vi "BKP_PowerSupplies1697B.vi"(4 "Error In":errorcluster, 7 "Command":T13) -> (0 "Error Out":errorcluster, 3 "Response":T11)   [LabVIEW 2018]
uses:
  MOKO_LabViewLibrary/MokoLowLevel/MokoLowLovelControl/MLLC_Command.ctl
  MOKO_LabViewLibrary/MokoLowLevel/MokoLowLovelControl/MLLC_Mode.ctl
  MOKO_LabViewLibrary/MokoLowLevel/MokoLowLovelControl/MLLC_Response.ctl
  MOKO_LabViewLibrary/MokoLowLevel/MokoLowLovelControl/MLLC_ConnectCluster.ctl
  MOKO_LabViewLibrary/MokoLowLevel/MokoLowLovelControl/MLLC_InterfaceType.ctl
  MOKO_LabViewLibrary/MokoLowLevel/MokoLowLovelControl/MLLC_OpenedSession.ctl
  MOKO_LabViewLibrary/MokoLowLevel/MokoLowLovelControl/MLLC_InterfaceSettings.ctl
  MOKO_LabViewLibrary/MokoLowLevel/MokoLowLovelControl/MLLC_InterfaceKind.ctl
  MOKO_LabViewLibrary/MokoLowLevel/MokoLowLovelControl/MLLC_DriverName.ctl
  MOKO_LabViewLibrary/MokoLowLevel/MokoLowLovelControl/MLLC_ResponseInit.ctl
  MOKO_LabViewLibrary/MokoLowLevel/MokoLowLovelControl/MLLC_Request.ctl
  MOKO_LabViewLibrary/MokoLowLevel/MokoLowLovelControl/MLLC_ErrorCode.ctl
  MOKO_LabViewLibrary/MokoLowLevel/MokoLowLovelControl/MLLC_Rs232Settings.ctl
panel:
  in  "Error Code":T1=5420
  in  "Request":T2="GETS"
  in  "ResponseInit":T3="OK"
  in  "Driver Name":T4="BK1697B"
  in  "Settings":T10={"Permanent data"={"Connect"={"InterfaceType"=enum."VISA", "OpenedSession"="", "InterfaceSettings"={"Interface"=enum."RS232", "EOS 4 read"=enum."CR (\\r)", "EOS 4 write"=enum."CR (\\r)", "TMO, ms"=2000, "Sett"=variant(cluster{"Baud Rate":u32, "Data Bits":u16, "Parity":u16, "Stop Bits":u16, "Flow Control":u16, "Eho":bool} {"Baud Rate"=75, "Data Bits"=0, "Parity"=0, "Stop Bits"=0, "Flow Control"=0, "Eho"=FALSE})}}}, "Saved Data"=variant}
  in  "Mode":T12=enum."Check"
  # "BK1697B"
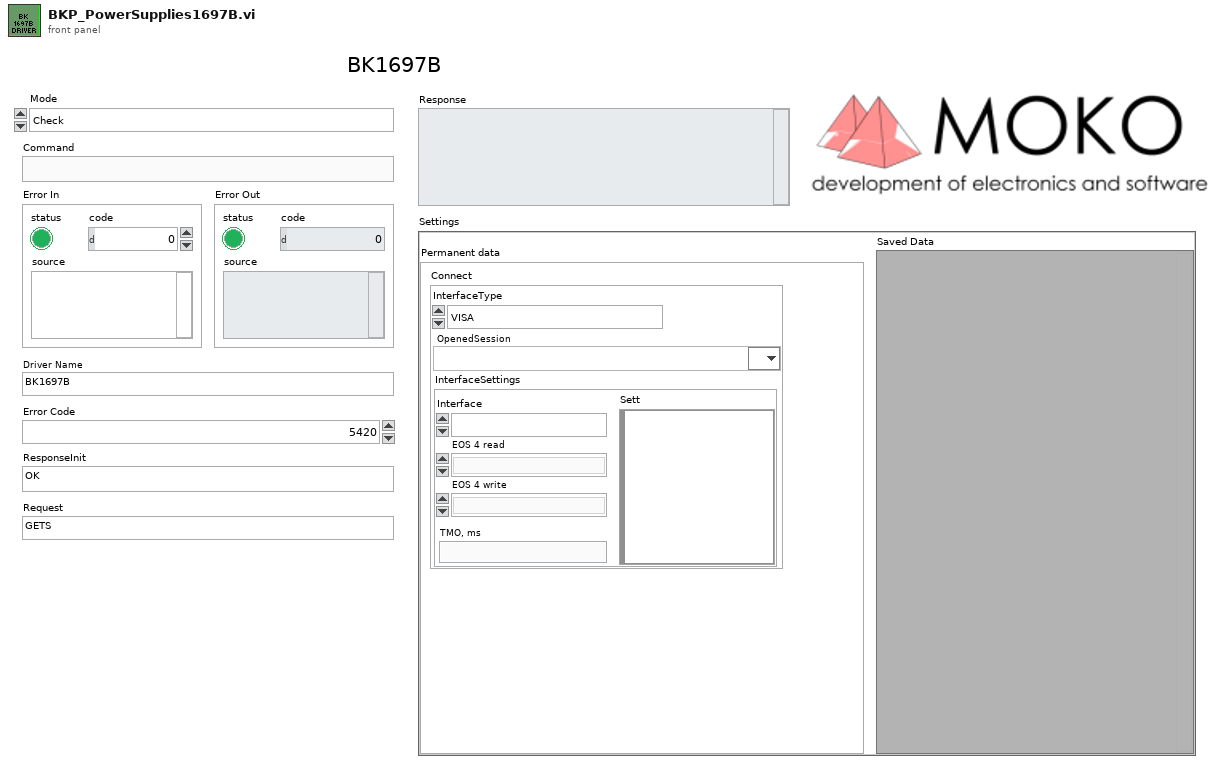
[diagram p1: front panel]
types:
  T1 = typedef "MLLC_ErrorCode.ctl" = u32
  T2 = typedef "MLLC_Request.ctl" = string
  T3 = typedef "MLLC_ResponseInit.ctl" = string
  T4 = typedef "MLLC_DriverName.ctl" = string
  T5 = typedef "MLLC_ConnectCluster.ctl" = cluster{"InterfaceType":T6, "OpenedSession":T7, "InterfaceSettings":T8}
  T6 = typedef "MLLC_InterfaceType.ctl" = enum16{"VISA", "Prologix USB-GPIB"}
  T7 = typedef "MLLC_OpenedSession.ctl" = refnum<visa-resource-name>
  T8 = typedef "MLLC_InterfaceSettings.ctl" = cluster{"Interface":T9, "EOS 4 read":enum16{"Default (=EOS 4 write)", "CR (\\r)", "LF (\\n)", "None"}, "EOS 4 write":enum16{"CR+LF (\\r\\n)", "CR (\\r)", "LF (\\n)", "None"}, "TMO, ms":i32, "Sett":variant}
  T9 = typedef "MLLC_InterfaceKind.ctl" = enum16{"RS232", "GPIB", "USB", "Ethernet", "another"}
  T10 = cluster{"Permanent data":cluster{"Connect":T5}, "Saved Data":variant}
  T11 = typedef "MLLC_Response.ctl" = string
  T12 = typedef "MLLC_Mode.ctl" = enum16{"get", "set", "close", "Init", "Check"}
  T13 = typedef "MLLC_Command.ctl" = string
  T14 = typedef "MLLC_Error.ctl" = errorcluster
  T15 = typedef "MLLC_Rs232Settings.ctl" = cluster{"Baud Rate":u32, "Data Bits":u16, "Parity":u16, "Stop Bits":u16, "Flow Control":u16, "Eho":bool, "Address":dbl}
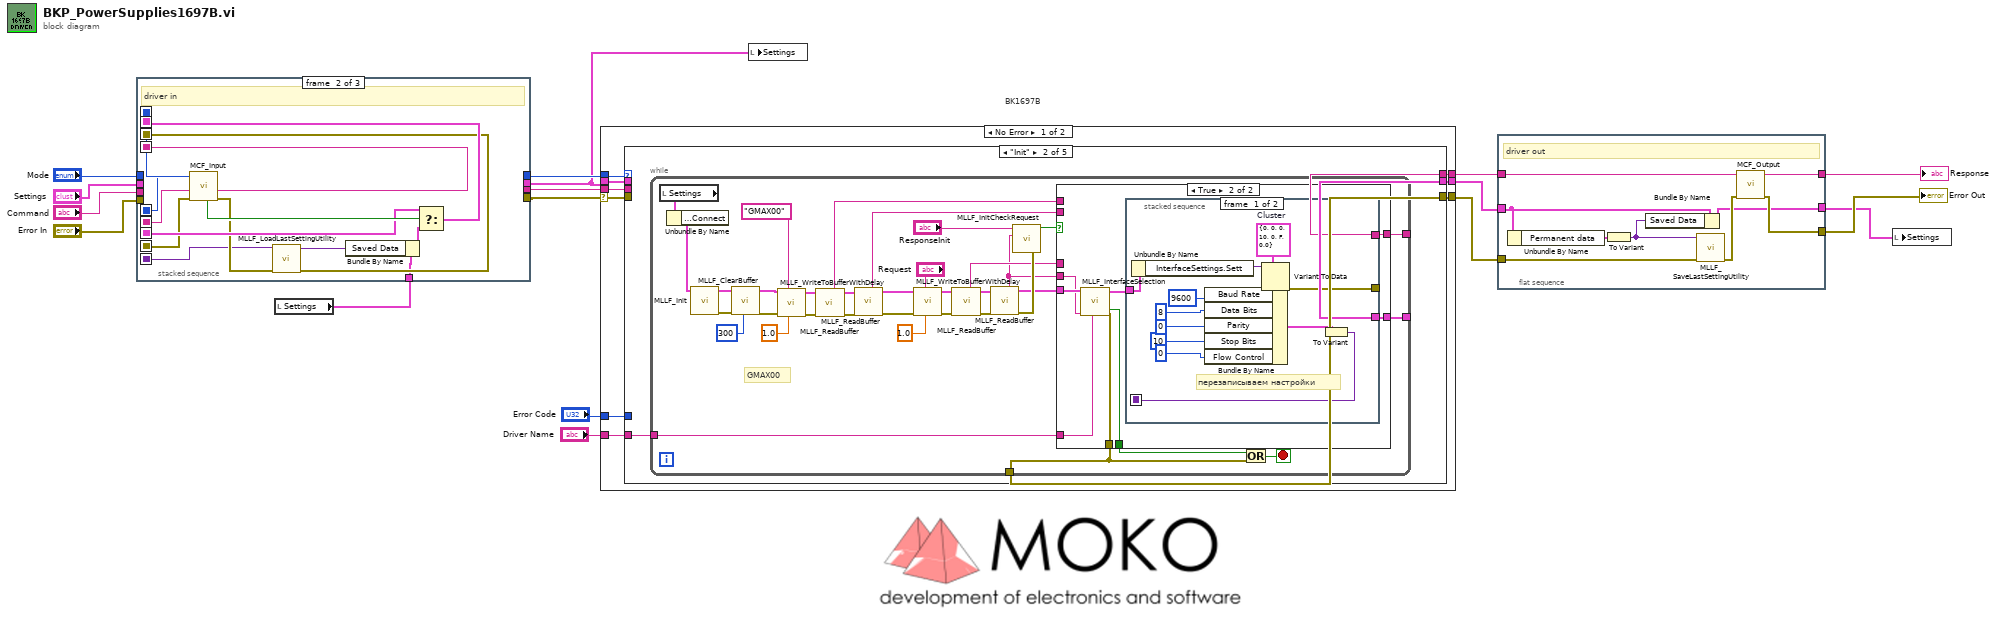
[diagram p0: block diagram]
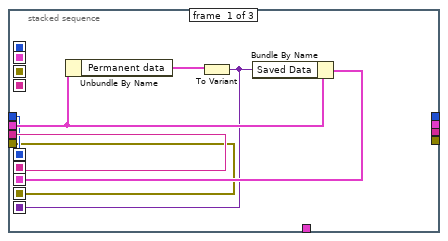
[diagram p2: hidden frame]
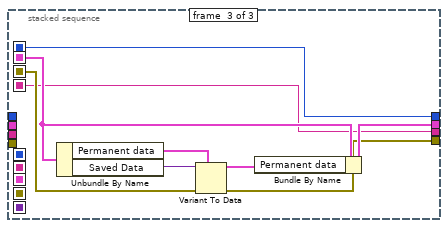
[diagram p3: hidden frame]
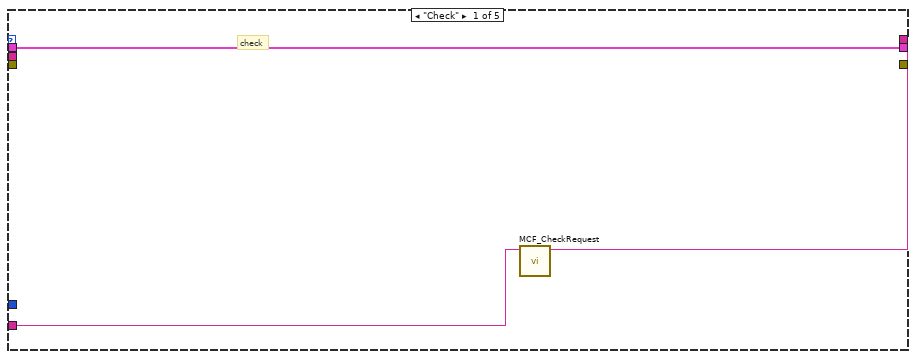
[diagram p4: hidden frame]
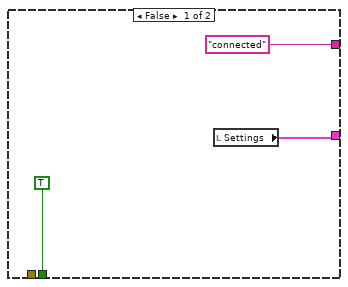
[diagram p5: hidden frame]
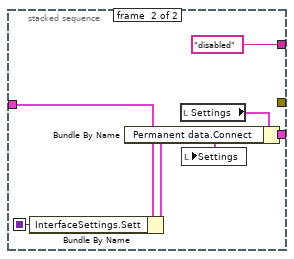
[diagram p6: hidden frame]
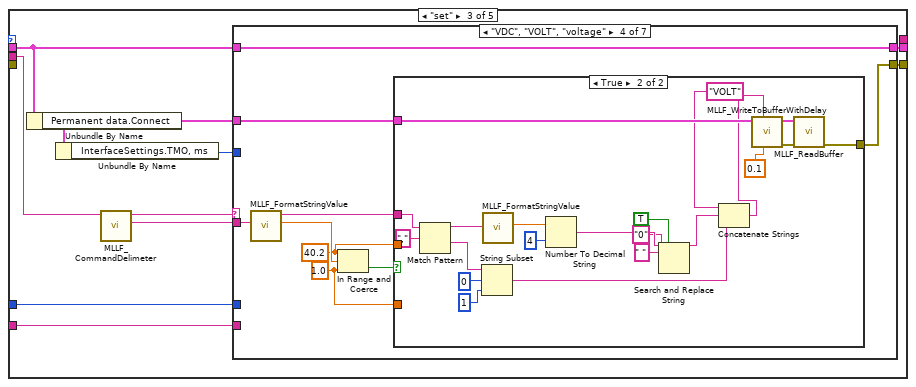
[diagram p7: hidden frame]
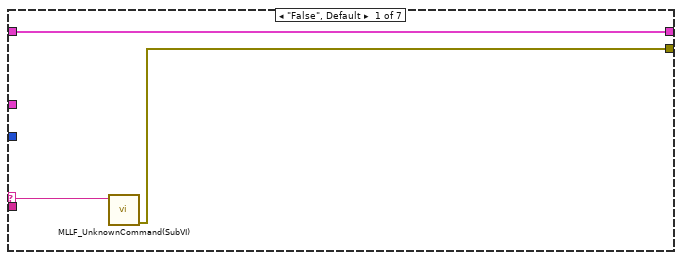
[diagram p8: hidden frame]
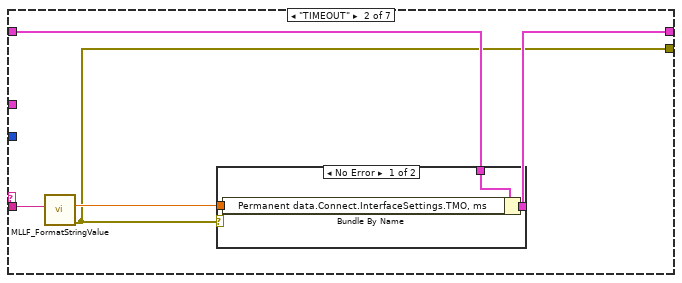
[diagram p9: hidden frame]
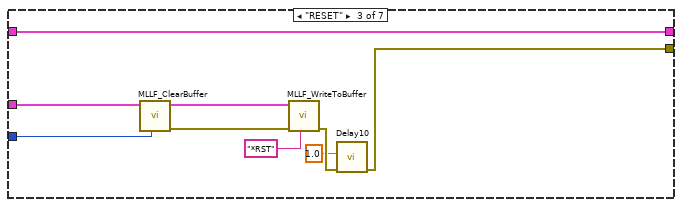
[diagram p11: hidden frame]
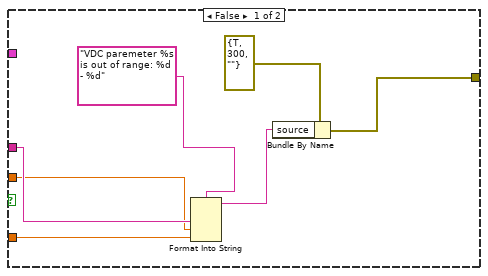
[diagram p12: hidden frame]
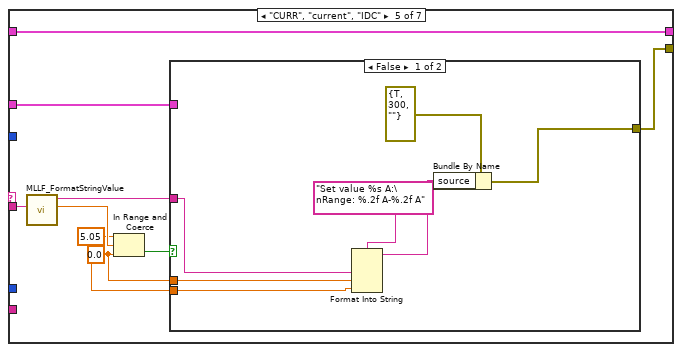
[diagram p13: hidden frame]
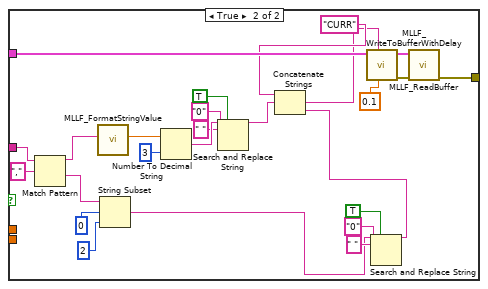
[diagram p14: hidden frame]
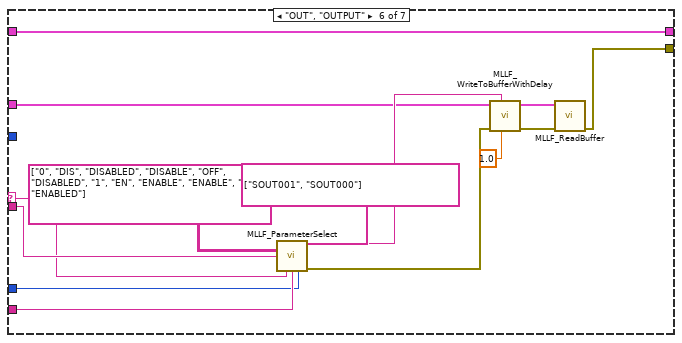
[diagram p15: hidden frame]
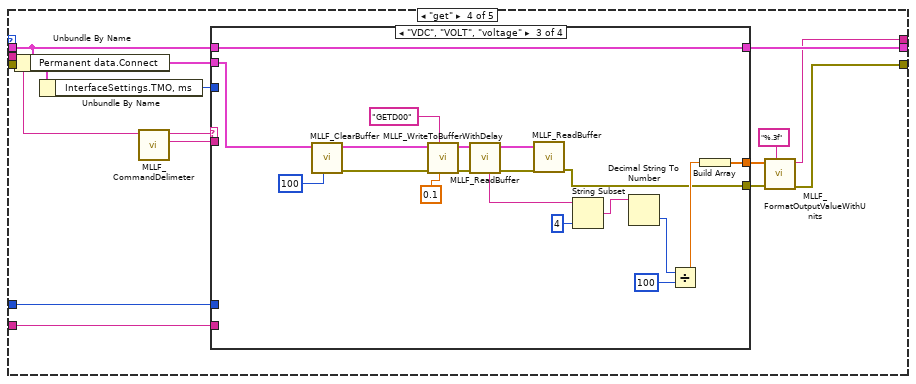
[diagram p17: hidden frame]
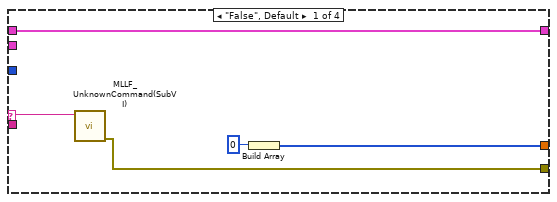
[diagram p18: hidden frame]
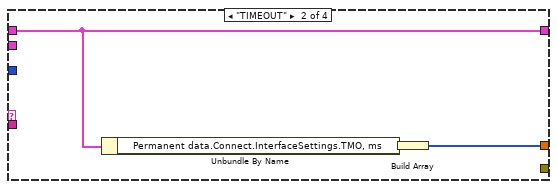
[diagram p19: hidden frame]
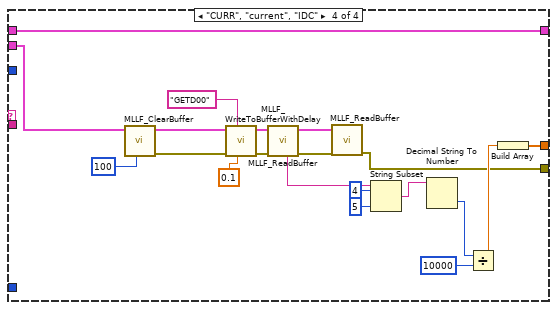
[diagram p20: hidden frame]
diagram:
  # "BK1697B"
  n1 = local read "Settings"() -> (w8:T10)
  n2 = stacked-sequence {
    seq-local: [w20 _ _] -> [_ w36 _]
    seq-local: [w19 _ _] -> [_ w37 _]
    seq-local: [w22 _ _] -> [_ w32 _]
    seq-local: [w18 _ _] -> [_ w31 _]
    seq-local: [w21 _ _] -> [_ w27 _]
    seq-local: [_ w28 _] -> [_ _ w44]
    seq-local: [_ w38 _] -> [_ _ w41]
    seq-local: [_ w35 _] -> [_ _ w40]
    seq-local: [_ w34 _] -> [_ _ w45]
    tunnel: "Command" -> [w20 _ _]
    tunnel: "Mode" -> [w19 _ _]
    tunnel: "Error In" -> [w18 _ _]
    tunnel: "Settings" -> [w23 _ _]
    tunnel: w8 -> [_ w26 _]
    tunnel: [_ _ w40] -> w10
    tunnel: [_ _ w43] -> w1
    tunnel: [_ _ w42] -> w9
    tunnel: [_ _ w41] -> w11
    frame #0 {
      n3 = Unbundle By Name(w23) -> ("Permanent data"=w24:cluster{"Connect":T5})
      n4 = To Variant(anything=w24) -> (Variant=w21:variant)
      n5 = Bundle By Name(cluster=w23, "Saved Data"=w21) -> (w22:T10)
    }
    frame #1 {
      # "driver in"
      n6 = call "MCF_Input.vi"("Error In"=w31, "Command in"=w36, "Mode in"=w37) -> ("Error Out"=w30:errorcluster, "Command out"=w35:string, "Mode out"=w38:T12, "Boolean"=w33:bool)  [unwired: 5 in]
      n7 = call "MLLF_LoadLastSettingUtility.vi"("Error In"=w30, "Save data in"=w27) -> ("Error Out"=w28:errorcluster, "Save data out"=w25:variant)  [unwired: 8 in]
      n8 = Bundle By Name(cluster=w26, "Saved Data"=w25) -> (w29:T10)
      n9 = Select(t=w32, s=w33, f=w29) -> (s? t:f=w34:T10)
    }
    frame #2 {
      n10 = Unbundle By Name(w45) -> ("Permanent data"=w46:cluster{"Connect":T5}, "Saved Data"=w39:variant)
      n11 = Variant To Data(error in=w44, type=w46, Variant=w39) -> (data=w47:cluster{"Connect":T5}, error out=w42:errorcluster)
      n12 = Bundle By Name(cluster=w45, "Permanent data"=w47) -> (w43:T10)
    }
  }
  n13 = case shown="No Error" w9 {
    selector: w9 -> [w52 w318]
    tunnel: [w54 w318] -> w5
    tunnel: w11 -> [w56 _]
    tunnel: [w55 _] -> w7
    tunnel: w10 -> [w53 _]
    tunnel: w1 -> [w49 w317]
    tunnel: "Error Code" -> [w51 _]
    tunnel: "Driver Name" -> [w50 _]
    tunnel: [w48 w317] -> w6
    frame No Error {
      n14 = case shown="\"Init\"" w56 {
        tunnel: [w57 w61 _ w253 "" ("Output String")] -> w55
        tunnel: [_ w63 w131 w254 w315] -> w54
        tunnel: w53 -> [_ _ w130 w259 _]
        tunnel: w52 -> [_ _ _ _ _]
        tunnel: w51 -> [_ _ w137 w263 _]
        tunnel: w50 -> [w58 w60 w134 w262 _]
        tunnel: w49 -> [w59 _ w136 w265 w314]
        tunnel: [w59 w62 w135 w264 w314] -> w48
        frame "Check" {
          # "check"
          n15 = call "MCF_CheckRequest.vi"("Driver Name"=w58) -> ("Output String"=w57:string)  [unwired: 9 in, 1 out]
        }
        frame "Init" {
          n16 = while {
            tunnel: [w92] -> w63
            tunnel: [w89] -> w62
            tunnel: [w88] -> w61
            tunnel: w60 -> [w77]
            stop <- w94 stop-if-true
            # "GMAX00"
            n17 = local read "Settings"() -> (w98:T10)
            n18 = Unbundle By Name(w98) -> ("Permanent data.Connect"=w95:T5)
            n19 = call "MLLF_Init.vi"("DriverConnect in"=w95) -> ("Error Out"=w80:errorcluster, "DriverConnect out"=w81:T5)  [unwired: 7 in]
            n20 = call "MLLF_ClearBuffer.vi"("Timeout(default = 300 ms)"=u32 300 ("Timeout"), "Error In"=w80, "DriverConnect in"=w81) -> ("Error Out"=w69:errorcluster, "DriverConnect out"=w70:T5)  [unwired: 5 in, 1 out]
            n21 = call "MLLF_WriteToBufferWithDelay.vi"("Delay Time ( 0,05 s)"=1.0 ("Delay Time (s)"), "Command"=T2 "GMAX00" ("Request 2"), "Error In"=w69, "DriverConnect in"=w70) -> ("Error Out"=w74:errorcluster, "DriverConnect out"=w72:T5)  [unwired: 6 in]
            n22 = call "MLLF_ReadBuffer.vi"("Error In"=w74, "DriverConnect in"=w72) -> ("Error Out"=w76:errorcluster, "DriverConnect out"=w75:T5, "String"=w66:string)  [unwired: 6 in]
            n23 = call "MLLF_ReadBuffer.vi"("Error In"=w76, "DriverConnect in"=w75) -> ("Error Out"=w67:errorcluster, "DriverConnect out"=w68:T5, "String"=w65:string)  [unwired: 6 in]
            n24 = call "MLLF_WriteToBufferWithDelay.vi"("Delay Time ( 0,05 s)"=1.0 ("Delay Time (s)"), "Command"="Request", "Error In"=w67, "DriverConnect in"=w68) -> ("Error Out"=w91:errorcluster, "DriverConnect out"=w97:T5)  [unwired: 6 in]
            n25 = call "MLLF_ReadBuffer.vi"("Error In"=w91, "DriverConnect in"=w97) -> ("Error Out"=w84:errorcluster, "DriverConnect out"=w85:T5, "String"=w78:string)  [unwired: 6 in]
            n26 = call "MLLF_ReadBuffer.vi"("Error In"=w84, "DriverConnect in"=w85) -> ("Error Out"=w83:errorcluster, "DriverConnect out"=w82:T5, "String"=w64:string)  [unwired: 6 in]
            n27 = call "MLLF_InitCheckRequest.vi"("error in (no error)"=w83, "Answer"=w64, "Response Init"="ResponseInit") -> ("Design"=w86:bool)  [unwired: 5 in, 3 out]
            n28 = case shown="True" w86 {
              tunnel: w82 -> [_ w108]
              tunnel: [TRUE w104] -> w93
              tunnel: [_ w109] -> w92
              tunnel: [w99 w106] -> w89
              tunnel: ["connected" w105] -> w88
              tunnel: w78 -> [_ _]
              tunnel: w77 -> [_ w103]
              tunnel: w66 -> [_ _]
              tunnel: w65 -> [_ _]
              tunnel: w64 -> [_ w102]
              frame False {
                n29 = local read "Settings"() -> (w99:T10)
              }
              frame True {
                n30 = call "MLLF_InterfaceSelection.vi"("Driver Name"=w103, "Answer:"=w102, "DriverConnect in"=w108) -> ("error out"=w109:T14, "DriverConnect out"=w107:T5, "stop init?"=w104:bool)  [unwired: 4 in, 2 out]
                n31 = stacked-sequence {
                  seq-local: [w112 _] -> [_ w126]
                  tunnel: w107 -> [w111 w123]
                  tunnel: [w113 _] -> _
                  tunnel: [_ w125] -> w106
                  tunnel: [_ "disabled"] -> w105
                  frame #0 {
                    w115 = T15 {"Baud Rate"=0, "Data Bits"=0, "Parity"=0, "Stop Bits"=10, "Flow Control"=0, "Eho"=FALSE, "Address"=0.0}  # Cluster
                    # "перезаписываем настройки"
                    n32 = Unbundle By Name(w111) -> ("InterfaceSettings.Sett"=w114:variant)
                    n33 = Variant To Data(type=w115, Variant=w114) -> (data=w116:T15, error out=w113:errorcluster)  [unwired: 1 in]
                    n34 = Bundle By Name(cluster=w116, "Baud Rate"=u32 9600, "Data Bits"=u16 8 ("Serial Settings:Data Bits"), "Parity"=u16 0 ("Serial Settings:Parity"), "Stop Bits"=u16 10 ("Serial Settings:Stop Bits"), "Flow Control"=u16 0 ("Serial Settings:Flow Control")) -> (w121:T15)
                    n35 = To Variant(anything=w121) -> (Variant=w112:variant)
                  }
                  frame #1 {
                    n36 = Bundle By Name(cluster=w123, "InterfaceSettings.Sett"=w126) -> (w122:T5)
                    n37 = local read "Settings"() -> (w127:T10)
                    n38 = Bundle By Name(cluster=w127, "Permanent data.Connect"=w122) -> (w125:T10)
                    n39 = local write "Settings"(w125) -> ()
                  }
                }
              }
            }
            n40 = Or(x=w93, y=w92) -> (x .or. y?=w94:bool)
          }
        }
        frame "set" {
          n41 = Unbundle By Name(w136) -> ("Permanent data.Connect"=w133:T5)
          n42 = Unbundle By Name(w133) -> ("InterfaceSettings.TMO, ms"=w132:i32)
          n43 = call "MLLF_CommandDelimeter.vi"("command with param"=w130) -> ("param 1"=w128:string, "command"=w129:string)  [unwired: 6 in, 3 out]
          n44 = case shown="\"VDC\", \"VOLT\", \"voltage\"" w129 {
            selector: w129 -> [w139 _ _ _ _ w240 _]
            tunnel: w128 -> [_ w143 _ w166 w203 w249 _]
            tunnel: w137 -> [_ _ _ _ _ w245 _]
            tunnel: w136 -> [w140 w144 w158 w167 w204 w250 w251]
            tunnel: [w140 w145 w158 w167 w204 w250 w251] -> w135
            tunnel: w133 -> [_ _ w156 w165 w202 w241 _]
            tunnel: w134 -> [_ _ _ _ _ w246 _]
            tunnel: w132 -> [_ _ w153 _ _ _ _]
            tunnel: [w138 w141 w150 w164 w201 w237 _] -> w131
            frame "False", Default {
              n45 = call "MLLF_UnknownCommand(SubVI).vi"("Unknown command"=w139) -> ("error out"=w138:errorcluster)  [unwired: 10 in]
            }
            frame "TIMEOUT" {
              n46 = call "MLLF_FormatStringValue.vi"("String Value"=w143) -> ("error out"=w141:T14, "number"=w142:dbl)  [unwired: 8 in, 1 out]
              n47 = case shown="No Error" w141 {
                tunnel: [w148 w149] -> w145
                tunnel: w144 -> [w147 w149]
                tunnel: w142 -> [w146 _]
                frame No Error {
                  n48 = Bundle By Name(cluster=w147, "Permanent data.Connect.InterfaceSettings.TMO, ms"=w146) -> (w148:T10)
                }
                frame Error {
                }
              }
            }
            frame "RESET" {
              n49 = call "MLLF_ClearBuffer.vi"("Timeout(default = 300 ms)"=w153, "DriverConnect in"=w156) -> ("Error Out"=w155:errorcluster, "DriverConnect out"=w154:T5)  [unwired: 6 in, 1 out]
              n50 = call "MLLF_WriteToBuffer.vi"("String"="*RST", "error in"=w155, "DriverConnect in"=w154) -> ("error out"=w152:T14)  [unwired: 5 in, 1 out]
              n51 = call "Delay10"("error in (no error)"=w152, "Delay Time (s)"=1.0) -> ("error out"=w150:errorcluster)  [unwired: 9 in]
            }
            frame "VDC", "VOLT", "voltage" {
              w160 = 1.0 ("lower limit")
              w159 = 40.2 ("upper limit")
              n52 = call "MLLF_FormatStringValue.vi"("String Value"=w166) -> ("number"=w162:dbl, "String Value Formated"=w163:T13)  [unwired: 8 in, 1 out]
              n53 = In Range and Coerce(upper limit=w159, x=w162, lower limit=w160) -> (In Range?=w161:bool)  [unwired: 1 out]
              n54 = case shown="True" w161 {
                tunnel: w165 -> [_ w192]
                tunnel: [w173 w191] -> w164
                tunnel: w163 -> [w172 w188]
                tunnel: w160 -> [w169 _]
                tunnel: w159 -> [w168 _]
                frame False {
                  n55 = Format Into String(format string="VDC paremeter %s is out of range: %d - %d", w172, w168, w169) -> (resulting string=w171:string)  [unwired: 2 in, 1 out]
                  n56 = Bundle By Name(cluster=errorcluster {"status"=TRUE, "code"=300, "source"=""} ("Error Out"), "source"=w171) -> (w173:errorcluster)
                }
                frame True {
                  n57 = Match Pattern(string=w188, regular expression=",") -> (before substring=w180:T13, after substring=w186:T13)  [unwired: 1 in, 2 out]
                  n58 = String Subset(string=w186, offset (0)=0, length (rest)=1 ("length (rest)")) -> (substring=w183:T13)
                  n59 = call "MLLF_FormatStringValue.vi"("String Value"=w180) -> ("number"=w182:dbl)  [unwired: 8 in, 2 out]
                  n60 = Number To Decimal String(number=w182, width (-)=i16 4) -> (decimal integer string=w179:string)
                  n61 = Search and Replace String(replace all?=TRUE ("replace all? (F)"), input string=w179, search string=" ", replace string="0" ("replace string (\"\")")) -> (result string=w176:string)  [unwired: 4 in, 3 out]
                  n62 = Concatenate Strings(T13 "VOLT" ("Command"), w176, w183) -> (w189:string)
                  n63 = call "MLLF_WriteToBufferWithDelay.vi"("Delay Time ( 0,05 s)"=0.1 ("Delay Time (s)"), "Command"=w189, "DriverConnect in"=w192) -> ("Error Out"=w194:errorcluster, "DriverConnect out"=w195:T5)  [unwired: 7 in]
                  n64 = call "MLLF_ReadBuffer.vi"("Error In"=w194, "DriverConnect in"=w195) -> ("Error Out"=w191:errorcluster)  [unwired: 6 in, 2 out]
                }
              }
            }
            frame "CURR", "current", "IDC" {
              w197 = 0.0 ("lower limit")
              w196 = 5.05 ("upper limit")
              n65 = call "MLLF_FormatStringValue.vi"("String Value"=w203) -> ("number"=w199:dbl, "String Value Formated"=w200:T13)  [unwired: 8 in, 1 out]
              n66 = In Range and Coerce(upper limit=w196, x=w199, lower limit=w197) -> (In Range?=w198:bool)  [unwired: 1 out]
              n67 = case shown="False" w198 {
                tunnel: w202 -> [_ w233]
                tunnel: [w210 w232] -> w201
                tunnel: w200 -> [w208 w229]
                tunnel: w197 -> [w206 _]
                tunnel: w196 -> [w205 _]
                frame False {
                  n68 = Format Into String(format string="Set value %s A:\nRange: %.2f A-%.2f A", w208, w206, w205) -> (resulting string=w207:string)  [unwired: 2 in, 1 out]
                  n69 = Bundle By Name(cluster=errorcluster {"status"=TRUE, "code"=300, "source"=""} ("Error Out"), "source"=w207) -> (w210:errorcluster)
                }
                frame True {
                  n70 = Match Pattern(string=w229, regular expression=",") -> (before substring=w222:T13, after substring=w227:T13)  [unwired: 1 in, 2 out]
                  n71 = call "MLLF_FormatStringValue.vi"("String Value"=w222) -> ("number"=w224:dbl)  [unwired: 8 in, 2 out]
                  n72 = String Subset(string=w227, offset (0)=0, length (rest)=2 ("length (rest)")) -> (substring=w213:T13)
                  n73 = Number To Decimal String(number=w224, width (-)=i16 3) -> (decimal integer string=w221:string)
                  n74 = Search and Replace String(replace all?=TRUE ("replace all? (F)"), input string=w221, search string=" ", replace string="0" ("replace string (\"\")")) -> (result string=w218:string)  [unwired: 4 in, 3 out]
                  n75 = Search and Replace String(replace all?=TRUE ("replace all? (F)"), input string=w213, search string=" ", replace string="0" ("replace string (\"\")")) -> (result string=w212:string)  [unwired: 4 in, 3 out]
                  n76 = Concatenate Strings(T13 "CURR" ("Command"), w218, w212) -> (w230:string)
                  n77 = call "MLLF_WriteToBufferWithDelay.vi"("Delay Time ( 0,05 s)"=0.1 ("Delay Time (s)"), "Command"=w230, "DriverConnect in"=w233) -> ("Error Out"=w235:errorcluster, "DriverConnect out"=w236:T5)  [unwired: 7 in]
                  n78 = call "MLLF_ReadBuffer.vi"("Error In"=w235, "DriverConnect in"=w236) -> ("Error Out"=w232:errorcluster)  [unwired: 6 in, 2 out]
                }
              }
            }
            frame "OUT", "OUTPUT" {
              n79 = call "MLLF_ParameterSelect.vi"("Command to equipment"=string[] ["SOUT001", "SOUT000"] ("Names"), "Names"=string[][] [["0", "DIS", "DISABLED", "DISABLE", "OFF", "DISABLED"], ["1", "EN", "ENABLE", "ENABLE", "ON", "ENABLED"]], "Input"=w249, "Command"=w240, "Driver Name"=w246, "Error Code"=w245) -> ("Choice"=w242:string, "Error Out"=w243:errorcluster)  [unwired: 8 in]
              n80 = call "MLLF_WriteToBufferWithDelay.vi"("Delay Time ( 0,05 s)"=1.0 ("Delay Time (s)"), "Command"=w242, "Error In"=w243, "DriverConnect in"=w241) -> ("Error Out"=w239:errorcluster, "DriverConnect out"=w238:T5)  [unwired: 6 in]
              n81 = call "MLLF_ReadBuffer.vi"("Error In"=w239, "DriverConnect in"=w238) -> ("Error Out"=w237:errorcluster)  [unwired: 6 in, 2 out]
            }
            frame "****************************************************" {
            }
          }
        }
        frame "get" {
          n82 = Unbundle By Name(w265) -> ("Permanent data.Connect"=w256:T5)
          n83 = Unbundle By Name(w256) -> ("InterfaceSettings.TMO, ms"=w255:i32)
          n84 = call "MLLF_CommandDelimeter.vi"("command with param"=w259) -> ("param 1"=w257:string, "command"=w258:string)  [unwired: 6 in, 3 out]
          n85 = case shown="\"VDC\", \"VOLT\", \"voltage\"" w258 {
            selector: w258 -> [w267 _ _ _]
            tunnel: w257 -> [_ _ _ _]
            tunnel: [w266 _ w278 w298] -> w261
            tunnel: w263 -> [_ _ _ _]
            tunnel: [w270 w273 w292 w312] -> w264
            tunnel: w265 -> [w270 w273 w292 w312]
            tunnel: [w268 w271 w281 w301] -> w260
            tunnel: w256 -> [_ _ w276 w296]
            tunnel: w262 -> [_ _ _ _]
            tunnel: w255 -> [_ _ _ _]
            frame "False", Default {
              n86 = call "MLLF_UnknownCommand(SubVI).vi"("Unknown command"=w267) -> ("error out"=w266:errorcluster)  [unwired: 10 in]
              n87 = Build Array(0 ("TimeOut")) -> (w268:i32[])
            }
            frame "TIMEOUT" {
              n88 = Unbundle By Name(w273) -> ("Permanent data.Connect.InterfaceSettings.TMO, ms"=w272:i32)
              n89 = Build Array(w272) -> (w271:i32[])
            }
            frame "VDC", "VOLT", "voltage" {
              n90 = call "MLLF_ClearBuffer.vi"("Timeout(default = 300 ms)"=u32 100 ("Timeout"), "DriverConnect in"=w276) -> ("Error Out"=w274:errorcluster, "DriverConnect out"=w275:T5)  [unwired: 6 in, 1 out]
              n91 = call "MLLF_WriteToBufferWithDelay.vi"("Delay Time ( 0,05 s)"=0.1 ("Delay Time (s)"), "Command"=T13 "GETD00", "Error In"=w274, "DriverConnect in"=w275) -> ("Error Out"=w290:errorcluster, "DriverConnect out"=w291:T5)  [unwired: 6 in]
              n92 = call "MLLF_ReadBuffer.vi"("Error In"=w290, "DriverConnect in"=w291) -> ("Error Out"=w280:errorcluster, "DriverConnect out"=w279:T5, "String"=w287:string)  [unwired: 6 in]
              n93 = call "MLLF_ReadBuffer.vi"("Error In"=w280, "DriverConnect in"=w279) -> ("Error Out"=w278:errorcluster)  [unwired: 6 in, 2 out]
              n94 = String Subset(string=w287, length (rest)=4 ("length (rest)")) -> (substring=w285:string)  [unwired: 1 in]
              n95 = Decimal String To Number(string=w285) -> (number=w284:i32)  [unwired: 2 in, 1 out]
              n96 = Divide(x=w284, y=100) -> (x/y=w282:dbl)
              n97 = Build Array(w282) -> (w281:dbl[])
            }
            frame "CURR", "current", "IDC" {
              n98 = call "MLLF_ClearBuffer.vi"("Timeout(default = 300 ms)"=u32 100 ("Timeout"), "DriverConnect in"=w296) -> ("Error Out"=w293:errorcluster, "DriverConnect out"=w294:T5)  [unwired: 6 in, 1 out]
              n99 = call "MLLF_WriteToBufferWithDelay.vi"("Delay Time ( 0,05 s)"=0.1 ("Delay Time (s)"), "Command"=T13 "GETD00", "Error In"=w293, "DriverConnect in"=w294) -> ("Error Out"=w310:errorcluster, "DriverConnect out"=w311:T5)  [unwired: 6 in]
              n100 = call "MLLF_ReadBuffer.vi"("Error In"=w310, "DriverConnect in"=w311) -> ("Error Out"=w300:errorcluster, "DriverConnect out"=w299:T5, "String"=w307:string)  [unwired: 6 in]
              n101 = call "MLLF_ReadBuffer.vi"("Error In"=w300, "DriverConnect in"=w299) -> ("Error Out"=w298:errorcluster)  [unwired: 6 in, 2 out]
              n102 = String Subset(string=w307, offset (0)=4, length (rest)=5 ("length (rest)")) -> (substring=w305:string)
              n103 = Decimal String To Number(string=w305) -> (number=w304:i32)  [unwired: 2 in, 1 out]
              n104 = Divide(x=w304, y=10000) -> (x/y=w302:dbl)
              n105 = Build Array(w302) -> (w301:dbl[])
            }
          }
          n106 = call "MLLF_FormatOutputValueWithUnits.vi"("Format"=T13 "%.3f", "error in"=w261, "ValuesIn"=w260) -> ("error out"=w254:T14, "Result string"=w253:T13)  [unwired: 7 in]
        }
        frame "close" {
          n107 = Unbundle By Name(w314) -> ("Permanent data.Connect.OpenedSession"=w316:T7)
          n108 = VISA Close(VISA resource name=w316) -> (error out=w315:errorcluster)  [unwired: 1 in]
        }
      }
    }
    frame Error {
    }
  }
  n109 = local write "Settings"(w1) -> ()
  n110 = flat-sequence {
    tunnel: [w327] -> w4
    tunnel: [w326] -> w3
    tunnel: w7 -> [w325]
    tunnel: w5 -> [w324]
    tunnel: w6 -> [w320]
    tunnel: [w322] -> w2
    frame #0 {
      # "driver out"
      n111 = Unbundle By Name(w320) -> ("Permanent data"=w319:cluster{"Connect":T5})
      n112 = To Variant(anything=w319) -> (Variant=w321:variant)
      n113 = Bundle By Name(cluster=w320, "Saved Data"=w321) -> (w322:T10)
      n114 = call "MLLF_SaveLastSettingUtility.vi"("error in"=w324, "Saved Data"=w321) -> ("error out"=w323:T14)  [unwired: 8 in, 1 out]
      n115 = call "MCF_Output.vi"("Error In"=w323, "Input"=w325) -> ("Error Out"=w326:errorcluster, "Output"=w327:string)  [unwired: 8 in]
    }
  }
  n116 = local write "Settings"(w2) -> ()
  "Response" <- w4
  "Error Out" <- w3
